vi "Pad FXP Raw Data Array.vi"(2 "Cluster Bool Array in":bool[](array[boolean])) -> (0 "Cluster Bool Array out":bool[](array[boolean]), 1 "Size (bytes)":i32)   [LabVIEW 2019, in "FPGA Register IO.lvlib"]
uses:
  FPGA Register IO.lvlib
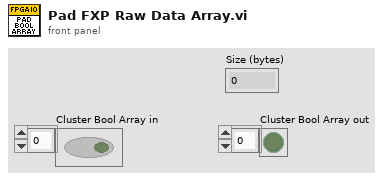
[diagram p1: front panel]
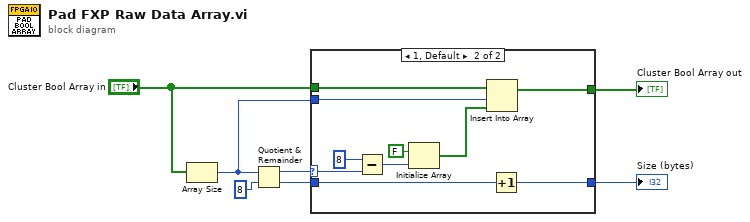
[diagram p0: block diagram]
diagram:
  n1 = Array Size(array="Cluster Bool Array in") -> (size(s)=w4:i32)
  n2 = Quotient & Remainder(x=w4, y=8) -> (x-y*floor(x/y)=w7:i32, floor(x/y)=w2:i32)
  n3 = case shown="1, Default" w7 {
    selector: w7 -> [_ w19]
    tunnel: "Cluster Bool Array in" -> [w9 w15]
    tunnel: w4 -> [_ w13]
    tunnel: [w9 w12] -> w3
    tunnel: w2 -> [w8 w11]
    tunnel: [w8 w10] -> w1
    frame 0 {
    }
    frame 1, Default {
      n4 = Subtract(x=8, y=w19) -> (x-y=w16:i32)
      n5 = Initialize Array(FALSE, w16) -> (w14:bool[])
      n6 = Insert Into Array(array=w15, index=w13, new element=w14) -> (w12:bool[])
      n7 = Increment(x=w11) -> (x+1=w10:i32)
    }
  }
  "Cluster Bool Array out" <- w3
  "Size (bytes)" <- w1
